vi "Get List of All VIs in Memory.vi"() -> ()   [LabVIEW 2014]
panel:
  in  "stop":bool
  out "Array":path[](array[path])
  out "VI number":i32
  out "error out":errorcluster
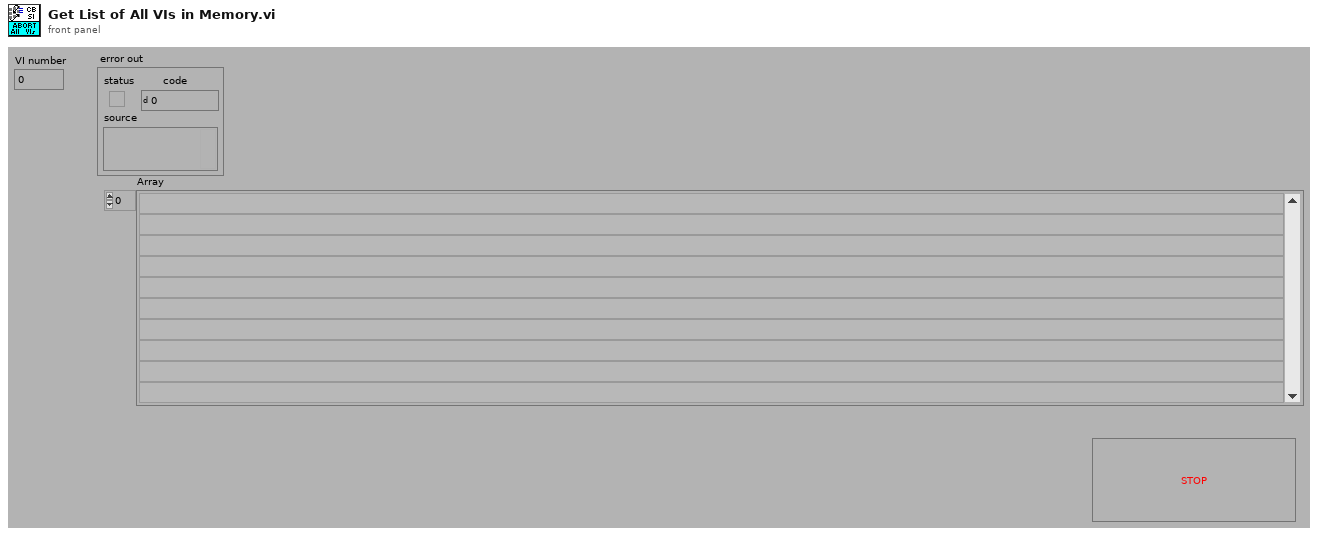
[diagram p1: front panel]
types:
  T1 = enum32{"Bad", "Idle", "Run top level", "Running"}
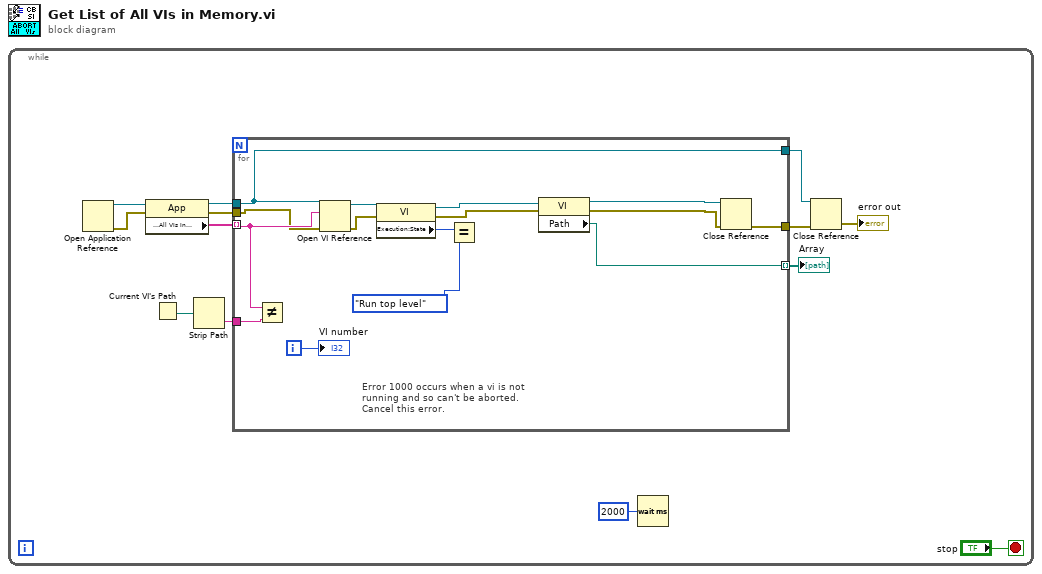
[diagram p0: block diagram]
diagram:
  n1 = while {
    stop <- "stop" stop-if-true
    n2 = Open Application Reference() -> (0:w10:errorcluster, 3:w13:refnum<vi>)  [unwired: 1 in, 3 out]
    n3 = property class="App"(reference=w13, error in=w10) -> (reference out=w11:refnum<vi>, error out=w5:errorcluster, "Application:All VIs In Memory"=w12:string[])
    n4 = Current VI's Path() -> (path=w7:path)
    n5 = Strip Path(path=w7) -> (name=w6:string)  [unwired: 1 out]
    n6 = for {
      tunnel: w12 -> [w26] mode=indexing
      tunnel: w11 -> [w28]
      tunnel: [w28] -> w8
      tunnel: w6 -> [w25]
      tunnel: w5 -> [w24]
      tunnel: [w23] -> w4
      tunnel: [w22] -> w3 mode=indexing
      i -> [w27]
      # "Error 1000 occurs when a vi is not\nrunning and so can't be aborted.  \nCancel this error."
      n7 = Not Equal?(x=w26, y=w25) -> ()  [unwired: 1 out]
      n8 = Open VI Reference(application reference (local)=w28, vi path=w26, error in (no error)=w24) -> (vi reference=w19:refnum<vi>, error out=w18:errorcluster)  [unwired: 3 out]
      n9 = property class="VI"(reference=w19, error in=w18) -> (reference out=w15:refnum<vi>, error out=w14:errorcluster, "Execution:State"=w17:T1)
      n10 = Equal?(x=w17, y=T1."Run top level" ("Execution:State")) -> ()  [unwired: 1 out]
      n11 = property class="VI"(reference=w15, error in=w14) -> (reference out=w20:refnum<vi>, error out=w21:errorcluster, "Path"=w22:path)
      n12 = Close Reference(reference=w20, error in (no error)=w21) -> (error out=w23:errorcluster)
      "VI number" <- w27
    }
    "Array" <- w3
    n13 = Wait (ms)(milliseconds to wait=u32 2000) -> ()  [unwired: 1 out]
    n14 = Close Reference(reference=w8, error in (no error)=w4) -> (error out=→"error out":errorcluster)
  }
